vi "lab3iii.vi"() -> ()   [LabVIEW 2020]
uses:
  <vilib>/addons/Control Design/_Model Construction/Model Creation.llb/CD Construct Transfer Function Model.vi
  <vilib>/addons/Control Design/_Model Construction/Model Creation.llb/Model Creation SubVI/cd_Create Transfer Function Model.vi
  <vilib>/addons/Control Design/_Model Interconnection/Model Interconnection.llb/Model Interconnection SubVI/cd_Series (TF and TF).vi
  <vilib>/addons/Control Design/_Model Interconnection/Model Interconnection.llb/Model Interconnection SubVI/cd_Feedback (TF and TF).vi
  <vilib>/addons/Control Design/_Model Conversions/Model Type.llb/Model Conversion SubVI/cd_Convert Transfer Function to Zero-Pole-Gain Model.vi
  <vilib>/addons/Control Design/_Utility/Model Viewer.llb/Model Viewer SubVI/cd_Draw Zero-Pole-Gain Equation (ZPK).vi
  <vilib>/addons/Control Design/_Utility/Model Viewer.llb/Model Viewer SubVI/cd_Draw Transfer Function Equation (TF).vi
  <vilib>/addons/Control Design/_Model Construction/NI_LinSys_Model Creation.lvlib
  <vilib>/addons/Control Design/_Model Interconnection/NI_CD_Model Interconnection.lvlib
  <vilib>/addons/Control Design/_Utility/NI_CD_Model Viewer.lvlib
  <vilib>/addons/Control Design/_Model Conversions/NI_CD_Model Type.lvlib
panel:
  out "Pole-Zero-Gain Model":picture
  out "Transfer function G(s)":picture
  in  "Numerator 10":dbl[](array[numeric]) format="%#.5g"
  in  "Denominator 10":dbl[](array[numeric]) format="%#.5g"
  in  "Numerator 9":dbl[](array[numeric]) format="%#.5g"
  in  "Denominator 9":dbl[](array[numeric]) format="%#.5g"
  in  "Numerator 8":dbl[](array[numeric]) format="%#.5g"
  in  "Denominator 8":dbl[](array[numeric]) format="%#.5g"
  in  "Numerator 7":dbl[](array[numeric]) format="%#.5g"
  in  "Denominator 7":dbl[](array[numeric]) format="%#.5g"
  in  "Numerator 6":dbl[](array[numeric]) format="%#.5g"
  in  "Denominator 6":dbl[](array[numeric]) format="%#.5g"
  in  "Numerator 5":dbl[](array[numeric]) format="%#.5g"
  in  "Denominator 5":dbl[](array[numeric]) format="%#.5g"
  in  "Numerator 4":dbl[](array[numeric]) format="%#.5g"
  in  "Denominator 4":dbl[](array[numeric]) format="%#.5g"
  in  "Numerator 3":dbl[](array[numeric]) format="%#.5g"
  in  "Denominator 3":dbl[](array[numeric]) format="%#.5g"
  in  "Numerator 2":dbl[](array[numeric]) format="%#.5g"
  in  "Denominator 2":dbl[](array[numeric]) format="%#.5g"
  in  "Denominator":dbl[](array[numeric]) format="%#.5g"
  in  "Numerator":dbl[](array[numeric]) format="%#.5g"
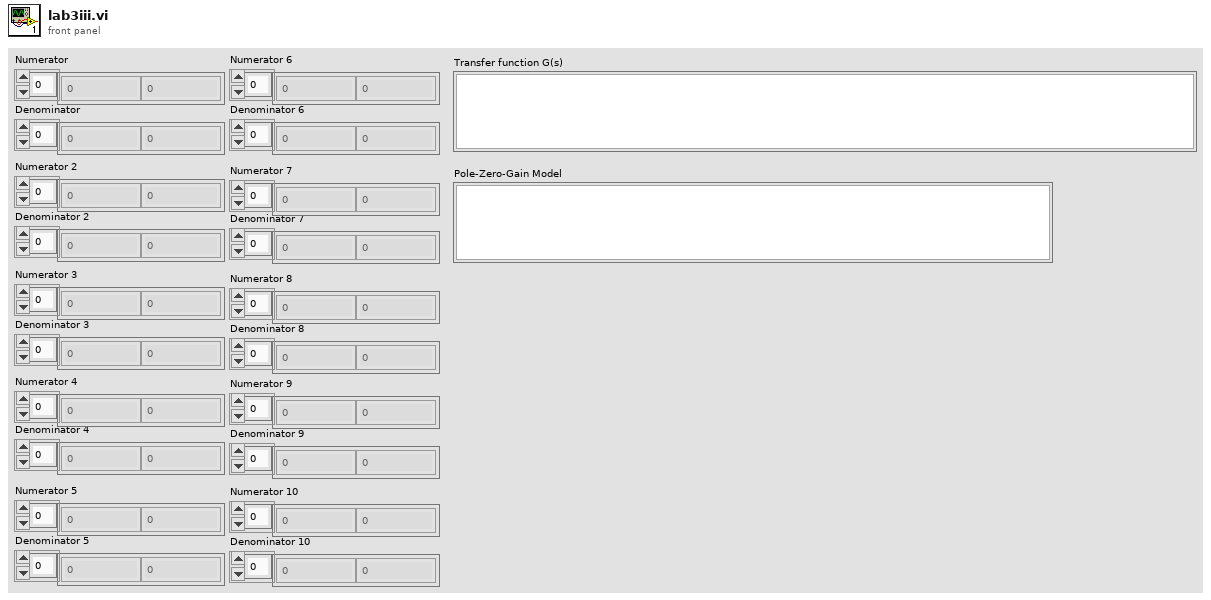
[diagram p1: front panel]
types:
  T1 = typedef "NI_LinSys_Model Typedefs.lvlib/CD Transfer Function Model (MIMO).ctl" = cluster{"properties":T2, "transfer function(s)":T3[][]}
  T2 = typedef "NI_LinSys_Model Typedefs.lvlib/CD General Elements.ctl" = cluster{"Model name":string, "Input names":string[], "Output names":string[], "Input Delays":dbl[], "Output Delays":dbl[], "Sampling Time":dbl, "Notes":string}
  T3 = typedef "NI_LinSys_Model Typedefs.lvlib/CD Transfer Function Model (SISO).ctl" = cluster{"Numerator":dbl[], "Denominator":dbl[], "delay":dbl}
  T4 = typedef "NI_LinSys_Model Typedefs.lvlib/CD Zero-Pole-Gain Model (MIMO).ctl" = cluster{"properties":T2, "zero-pole-gain(s)":T5[][]}
  T5 = typedef "NI_LinSys_Model Typedefs.lvlib/CD Zero-Pole-Gain Model (SISO).ctl" = cluster{"Gain":dbl, "Zeros":cdb[], "Poles":cdb[], "delay":dbl}
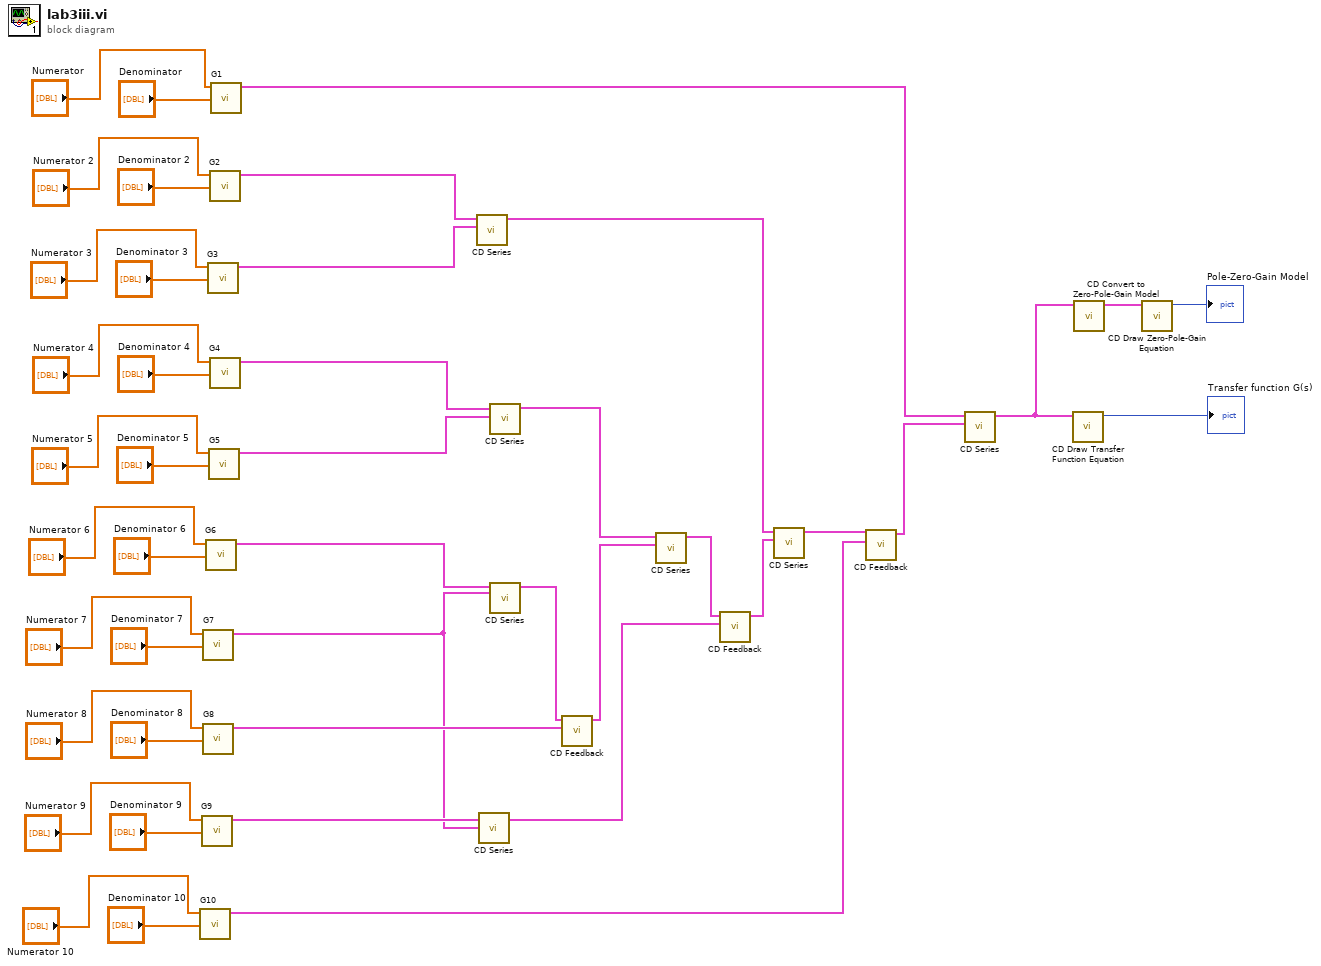
[diagram p0: block diagram]
diagram:
  n1 = call-poly "G10"("Denominator"="Denominator 10", "Numerator"="Numerator 10") -> ("Transfer Function Model"=w24:T1)  [unwired: 8 in, 1 out]
  n2 = call-poly "G9"("Denominator"="Denominator 9", "Numerator"="Numerator 9") -> ("Transfer Function Model"=w18:T1)  [unwired: 8 in, 1 out]
  n3 = call-poly "G7"("Denominator"="Denominator 7", "Numerator"="Numerator 7") -> ("Transfer Function Model"=w17:T1)  [unwired: 8 in, 1 out]
  n4 = call-poly "G8"("Denominator"="Denominator 8", "Numerator"="Numerator 8") -> ("Transfer Function Model"=w25:T1)  [unwired: 8 in, 1 out]
  n5 = call-poly "G6"("Denominator"="Denominator 6", "Numerator"="Numerator 6") -> ("Transfer Function Model"=w19:T1)  [unwired: 8 in, 1 out]
  n6 = call-poly "G3"("Denominator"="Denominator 3", "Numerator"="Numerator 3") -> ("Transfer Function Model"=w22:T1)  [unwired: 8 in, 1 out]
  n7 = call-poly "G5"("Denominator"="Denominator 5", "Numerator"="Numerator 5") -> ("Transfer Function Model"=w20:T1)  [unwired: 8 in, 1 out]
  n8 = call-poly "G2"("Denominator"="Denominator 2", "Numerator"="Numerator 2") -> ("Transfer Function Model"=w23:T1)  [unwired: 8 in, 1 out]
  n9 = call-poly "G4"("Denominator"="Denominator 4", "Numerator"="Numerator 4") -> ("Transfer Function Model"=w21:T1)  [unwired: 8 in, 1 out]
  n10 = call-poly "G1"("Denominator"="Denominator", "Numerator"="Numerator") -> ("Transfer Function Model"=w1:T1)  [unwired: 8 in, 1 out]
  n11 = call-poly <vilib>:"CD Series.vi"("Model 2"=w22, "Model 1"=w23) -> ("Series Model"=w11:T1)  [unwired: 8 in, 1 out]
  n12 = call-poly <vilib>:"CD Series.vi"("Model 2"=w17, "Model 1"=w18) -> ("Series Model"=w13:T1)  [unwired: 8 in, 1 out]
  n13 = call-poly <vilib>:"CD Series.vi"("Model 2"=w20, "Model 1"=w21) -> ("Series Model"=w14:T1)  [unwired: 8 in, 1 out]
  n14 = call-poly <vilib>:"CD Series.vi"("Model 2"=w17, "Model 1"=w19) -> ("Series Model"=w16:T1)  [unwired: 8 in, 1 out]
  n15 = call-poly <vilib>:"CD Feedback.vi"("Model 2"=w25, "Model 1"=w16) -> ("Closed-Loop Model"=w15:T1)  [unwired: 8 in, 1 out]
  n16 = call-poly <vilib>:"CD Series.vi"("Model 2"=w15, "Model 1"=w14) -> ("Series Model"=w12:T1)  [unwired: 8 in, 1 out]
  n17 = call-poly <vilib>:"CD Feedback.vi"("Model 2"=w13, "Model 1"=w12) -> ("Closed-Loop Model"=w10:T1)  [unwired: 8 in, 1 out]
  n18 = call-poly <vilib>:"CD Series.vi"("Model 2"=w10, "Model 1"=w11) -> ("Series Model"=w9:T1)  [unwired: 8 in, 1 out]
  n19 = call-poly <vilib>:"CD Feedback.vi"("Model 2"=w24, "Model 1"=w9) -> ("Closed-Loop Model"=w8:T1)  [unwired: 8 in, 1 out]
  n20 = call-poly <vilib>:"CD Series.vi"("Model 2"=w8, "Model 1"=w1) -> ("Series Model"=w6:T1)  [unwired: 8 in, 1 out]
  n21 = call-poly <vilib>:"CD Draw Transfer Function Equation.vi"("Transfer Function Model"=w6) -> ("Equation"=→"Transfer function G(s)":picture)  [unwired: 8 in, 2 out]
  n22 = call-poly <vilib>:"CD Convert to Zero-Pole-Gain Model.vi"("Transfer Function Model"=w6) -> ("Zero-Pole-Gain Model"=w5:T4)  [unwired: 9 in, 1 out]
  n23 = call-poly <vilib>:"CD Draw Zero-Pole-Gain Equation.vi"("Zero-Pole-Gain Model"=w5) -> ("Equation"=→"Pole-Zero-Gain Model":picture)  [unwired: 8 in, 2 out]
